vi "Complementary_Filter_LV_200hz.vi"(0 "Accel Data in":T1, 5 "Gyro Data in":T1, 7 "Dt( ms)":u32=5, 9 "Filter Time Constant":dbl=2.0, 11 "gyro_fsr":u32=1000) -> (4 "HP Gyro":dbl format="%0.2f", 6 "LP Accel":dbl format="%0.2f", 10 "Theta (rad)":dbl, 15 "Theta(deg)":dbl)   [LabVIEW 2014]
uses:
  <vilib>/Analysis/3filter.llb/Filter Passband Type.ctl
  <vilib>/ptbypt/NI_PtbyPt.lvlib
  <vilib>/Analysis/NI_AALBase.lvlib
panel:
  out "Dt":dbl
  out "gyro_fsr 2":u32=1000
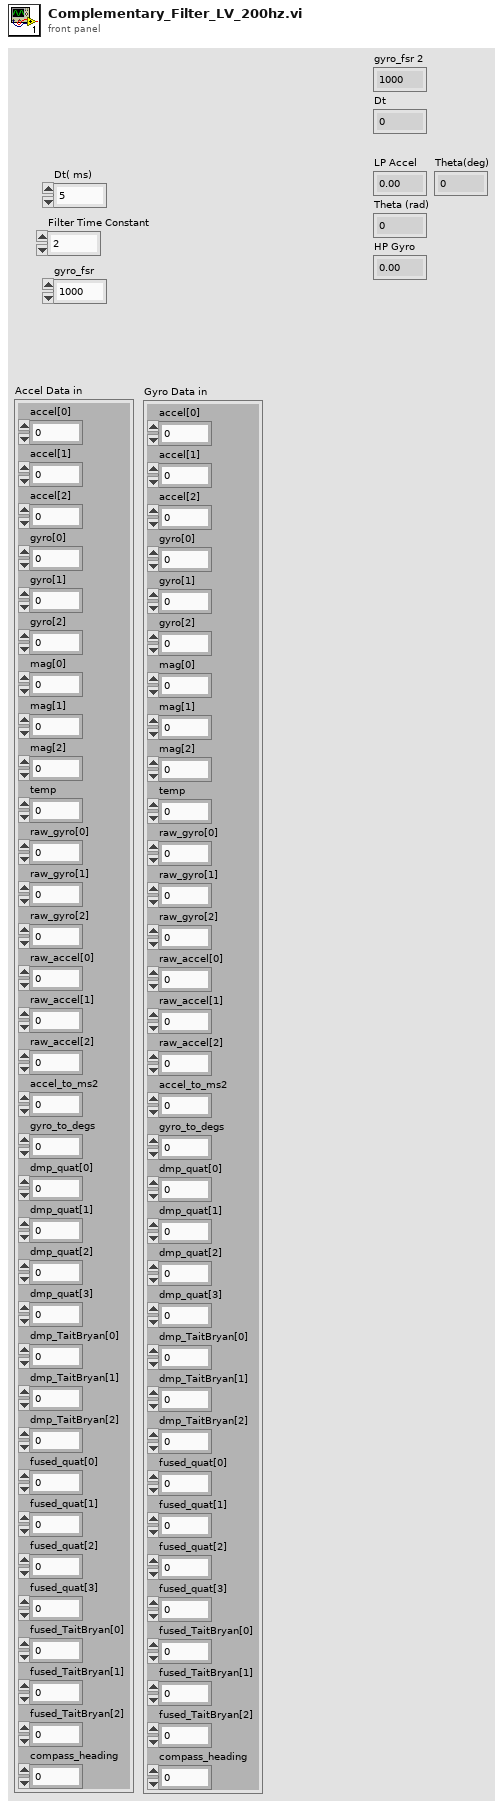
[diagram p1: front panel]
types:
  T1 = cluster{"accel[0]":sgl, "accel[1]":sgl, "accel[2]":sgl, "gyro[0]":sgl, "gyro[1]":sgl, "gyro[2]":sgl, "mag[0]":sgl, "mag[1]":sgl, "mag[2]":sgl, "temp":sgl, "raw_gyro[0]":i16, "raw_gyro[1]":i16, "raw_gyro[2]":i16, "raw_accel[0]":i16, "raw_accel[1]":i16, "raw_accel[2]":i16, "accel_to_ms2":sgl, "gyro_to_degs":sgl, "dmp_quat[0]":sgl, "dmp_quat[1]":sgl, "dmp_quat[2]":sgl, "dmp_quat[3]":sgl, "dmp_TaitBryan[0]":sgl, "dmp_TaitBryan[1]":sgl, "dmp_TaitBryan[2]":sgl, "fused_quat[0]":sgl, "fused_quat[1]":sgl, "fused_quat[2]":sgl, "fused_quat[3]":sgl, "fused_TaitBryan[0]":sgl, "fused_TaitBryan[1]":sgl, "fused_TaitBryan[2]":sgl, "compass_heading":sgl}
  T2 = typedef "NI_AALBase.lvlib/Filter Passband Type.ctl" = enum32{"Lowpass", "Highpass", "Bandpass", "Bandstop"}
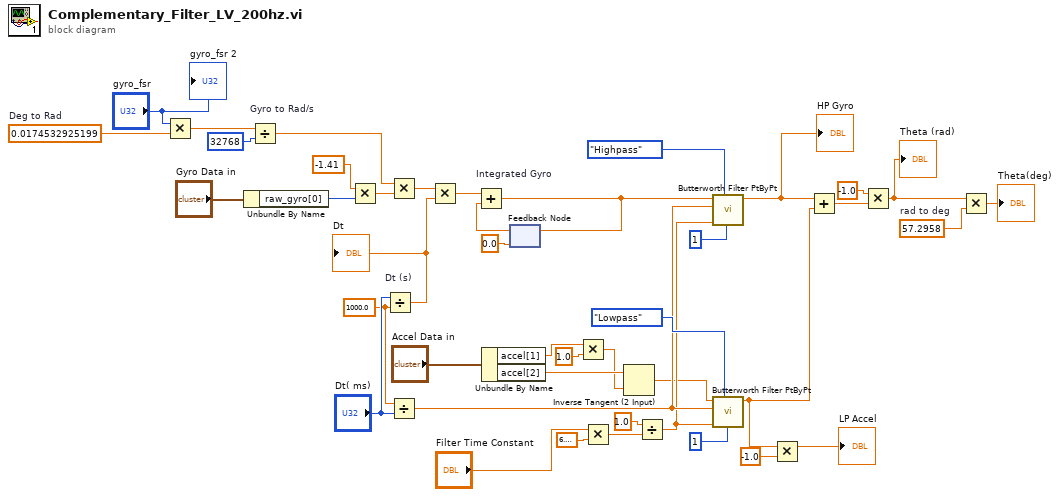
[diagram p0: block diagram]
diagram:
  w23 = 0.0174532925199  # Deg to Rad
  w6 = 1000.0 ("x")
  w31 = 57.2958  # rad to deg
  n1 = Multiply(x="gyro_fsr", y=w23) -> (x*y=w22:dbl)
  n2 = Unbundle By Name("Gyro Data in") -> ("raw_gyro[0]"=w40:i16)
  n3 = Divide "Gyro to Rad/s"(x=w22, y=u32 32768) -> (x/y=w19:dbl)
  n4 = Multiply(x=-1.41, y=w40) -> (x*y=w18:dbl)
  n5 = Divide "Dt (s)"(x="Dt( ms)", y=w6) -> (x/y=w5:dbl)
  "Dt" <- w5
  n6 = Multiply(x=w19, y=w18) -> (x*y=w9:dbl)
  n7 = Divide(x=w6, y="Dt( ms)") -> (x/y=w15:dbl)
  n8 = Multiply(x=w9, y=w5) -> (x*y=w8:dbl)
  n9 = Unbundle By Name("Accel Data in") -> ("accel[1]"=w42:sgl, "accel[2]"=w41:sgl)
  n10 = feedback #1(0.0) -> (w35:dbl)
  n11 = Add "Integrated Gyro"(x=w8, y=w35) -> (x+y=w17:dbl)
  n12 = feedback-in #1(w17) -> ()
  n13 = Multiply(x=w42, y=1.0) -> (x*y=w34:dbl)
  n14 = Multiply(x="Filter Time Constant", y=6.283185307179586) -> (x*y=w26:dbl)
  n15 = Inverse Tangent (2 Input)(1:w34, 2:w41) -> (0:w4:dbl)
  n16 = Divide(x=1.0, y=w26) -> (x/y=w14:dbl)
  n17 = call <vilib>:"Butterworth Filter PtByPt.vi"("order"=1, "filter type"=Filter_Passband_Type."Highpass", "low cutoff freq: fl"=w14, "sampling freq: fs"=w15, "x"=w17) -> ("Filtered x"=w3:dbl)  [unwired: 4 in, 1 out]
  "HP Gyro" <- w3
  n18 = call <vilib>:"Butterworth Filter PtByPt.vi"("order"=1, "filter type"=Filter_Passband_Type."Lowpass", "low cutoff freq: fl"=w14, "sampling freq: fs"=w15, "x"=w4) -> ("Filtered x"=w33:dbl)  [unwired: 4 in, 1 out]
  n19 = Multiply(x=w33, y=-1.0) -> (x*y=→"LP Accel":dbl)
  n20 = Add(x=w3, y=w33) -> (x+y=w32:dbl)
  n21 = Multiply(x=-1.0, y=w32) -> (x*y=w12:dbl)
  "Theta (rad)" <- w12
  n22 = Multiply(x=w12, y=w31) -> (x*y=→"Theta(deg)":dbl)
  "gyro_fsr 2" <- "gyro_fsr"
